vi "Run Display.vi"(8 "error in (no error)":errorcluster, 10 "Run?":bool) -> (0 "error out":errorcluster)   [LabVIEW 2016, in "AssertEngine.lvlib"]
uses:
  AssertEngine.lvlib
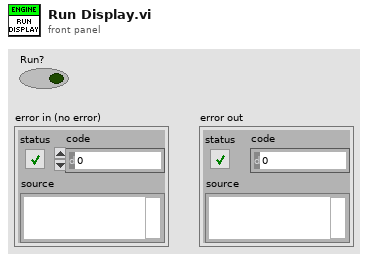
[diagram p1: front panel]
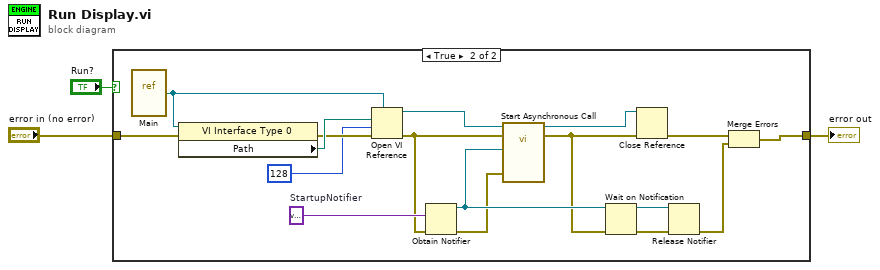
[diagram p0: block diagram]
diagram:
  n1 = case shown="True" "Run?" {
    tunnel: [w4 w9] -> w1
    tunnel: "error in (no error)" -> [w4 w16]
    frame False {
    }
    frame True {
      w17 = variant  # StartupNotifier
      n2 = vi-ref "Main.vi"() -> (w20:refnum<vi>)
      n3 = property class="VI Interface Type 0"(reference=w20, error in=w16) -> (error out=w19:errorcluster, "Path"=w21:path)  [unwired: 1 out]
      n4 = Open VI Reference(type specifier VI Refnum (for type only)=w20, vi path=w21, options=128, error in (no error)=w19) -> (vi reference=w18:refnum<vi>, error out=w15:errorcluster)  [unwired: 2 in]
      n5 = Obtain Notifier(notification data type=w17, error in (no error)=w15) -> (notifier out=w12:refnum<notifier>, error out=w11:errorcluster)  [unwired: 2 in, 1 out]
      n6 = call-by-ref "Start Asynchronous Call"(reference=w18, error in=w15, 8:"error in (no error)"=w11, "Startup Notifier"=w12) -> (reference out=w13:refnum<vi>, error out=w7:errorcluster)  [unwired: 10 in]
      n7 = Wait on Notification(notifier=w12, error in (no error)=w7) -> (notifier out=w10:refnum<notifier>, error out=w6:errorcluster)  [unwired: 2 in, 2 out]
      n8 = Close Reference(reference=w13, error in (no error)=w7) -> (error out=w14:errorcluster)
      n9 = Release Notifier(notifier=w10, error in (no error)=w6) -> (error out=w8:errorcluster)  [unwired: 1 in, 2 out]
      n10 = Merge Errors(w14, w8) -> (w9:errorcluster)
    }
  }
  "error out" <- w1
